vi "ScanningWaveform_v4 - Copy.vi"(0 "Vy-min":dbl, 1 "Vy-max":dbl, 2 "yPixels/tPixels":dbl, 3 "xPixels/rPixels":dbl, 4 "Vx-min":dbl, 5 "Vx-max":dbl, 6 "Drawing Mode":u16(ring) items=["Fill Rectangle", "Fill Circle", "Draw Freeform", "Fill Freeform"], 7 "Angle":dbl, 8 "Scanning Mode":u16(ring) items=["Raster", "Spiral"], 9 "AOrate":dbl, 10 "Points":cluster{"X":dbl, "Y":dbl}[](array[cluster])) -> (12 "numPixels":dbl, 13 "Y-WaveArray":dbl[](array[numeric]), 14 "P":dbl, 19 "X-WaveArray":dbl[](array[numeric]))   [LabVIEW 2013]
panel:
  out "min":dbl
  out "max":dbl
  out "Points 2":cluster{"R":dbl, "Theta":dbl}[](array[cluster])
  in  "yPixels/tPixels 2":dbl
  in  "xPixels/rPixels 2":dbl
  out "X-Y Graph":cluster{dbl[], dbl[]}(graph)
  out "flyback time (us)":dbl
  out "Y Graph":dbl[](graph)
  out "X Graph":dbl[](graph)
  out "C":dbl
  out "Sx":dbl
  out "S":dbl
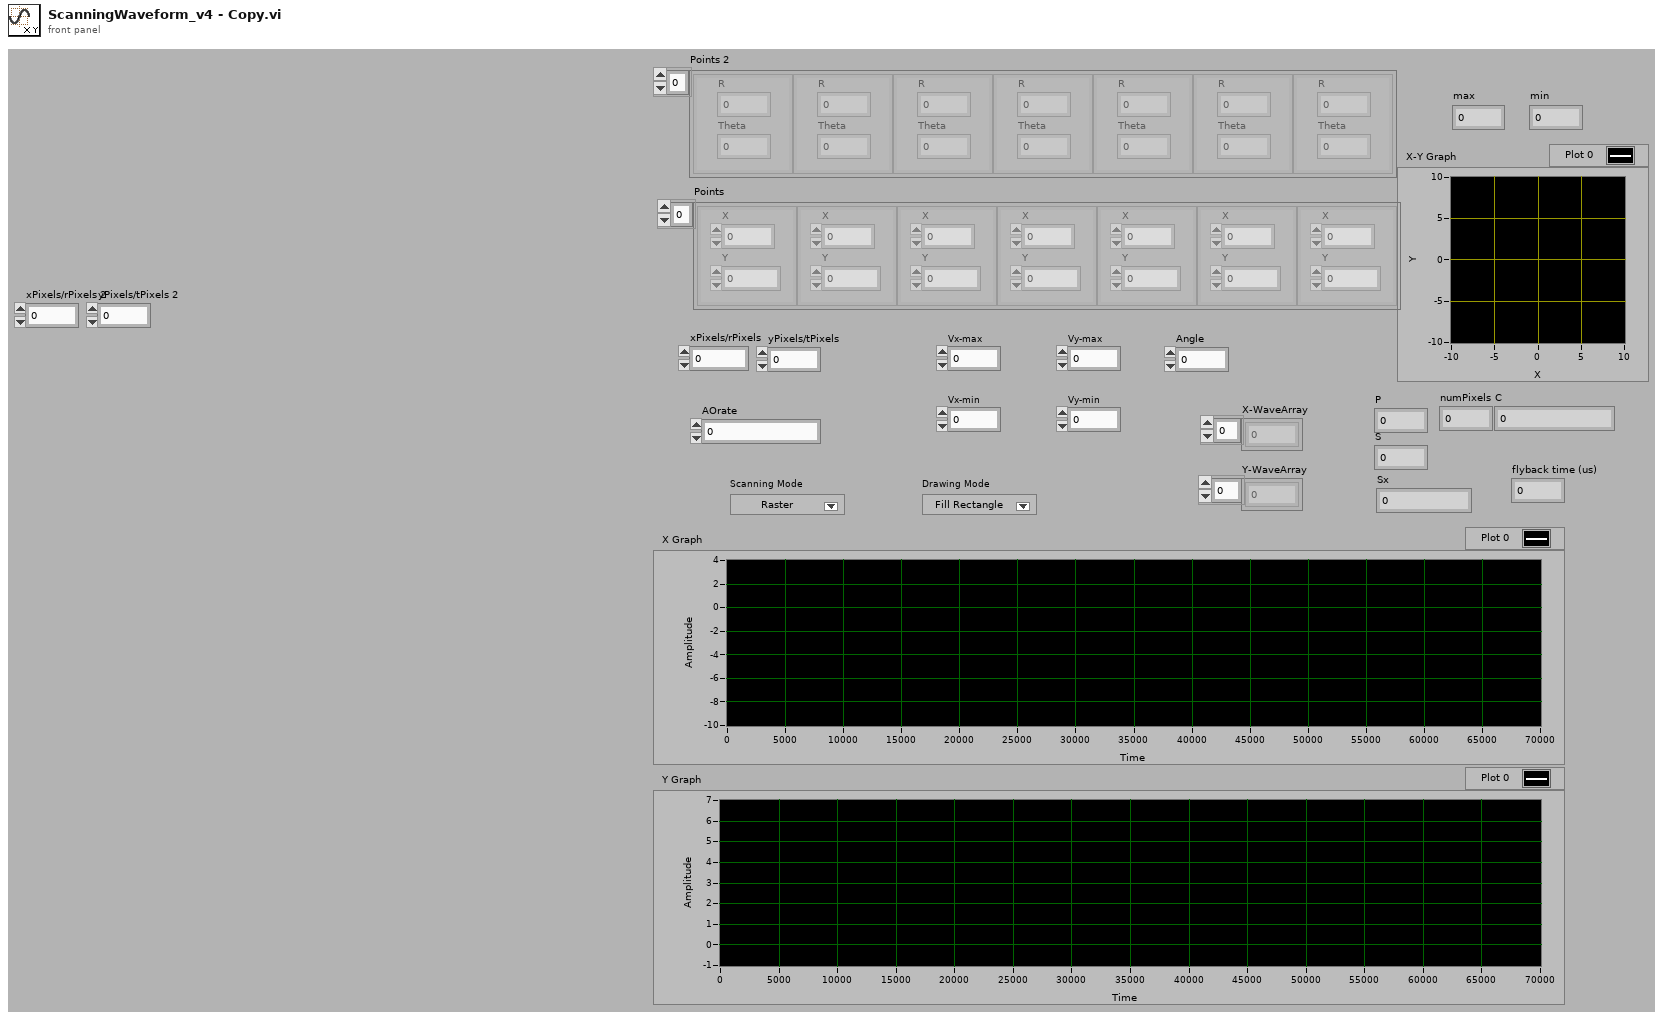
[diagram p1: front panel]
types:
  T1 = cluster{"Xpixels":i32, "Vx-min ref":dbl, "Vx-max ref":dbl, "Ypixels":i32, "Vy-min ref":dbl, "Vy-max ref":dbl, "srate":dbl, "type":string, "date":string, "time":string, "Colormap":u16, "square pixels":bool, "square matrix":bool, "Xpixels Img":i32, "Vx-min Img":dbl, "VX-max Img":dbl, "Ypixels Img":i32, "Vy-min Img":dbl, "Vy-max Img ":dbl, "autoshutter":bool, "P":dbl, "sAOxy":i32, "finite":bool, "cont":bool, "wavdet":bool, "measpoints":i32, "avpp":i32, "bufferAO":i32, "bufferAI":i32, "CH1":bool, "CH2":bool, "X":bool, "Y":bool, "timeout":dbl, "starttick":u32, "waveform":path, "Vy-ref":dbl, "Vx-ref":dbl, "refreshrate":dbl, "refreshbuffer":i32, "tt_cycles":i32, "motorref":refnum<k7>, "mirrorswitch":refnum<k7>, "sample mode":i32, "Ip":bool, "Vp":bool, "sampletreshold":dbl, "maxbufferAI":i32, "Angle Img":dbl, "Drawing Mode":u16, "Scanning Mode":u16}
  T2 = cluster{cluster{dbl, dbl}[], cluster{dbl, dbl}[]}
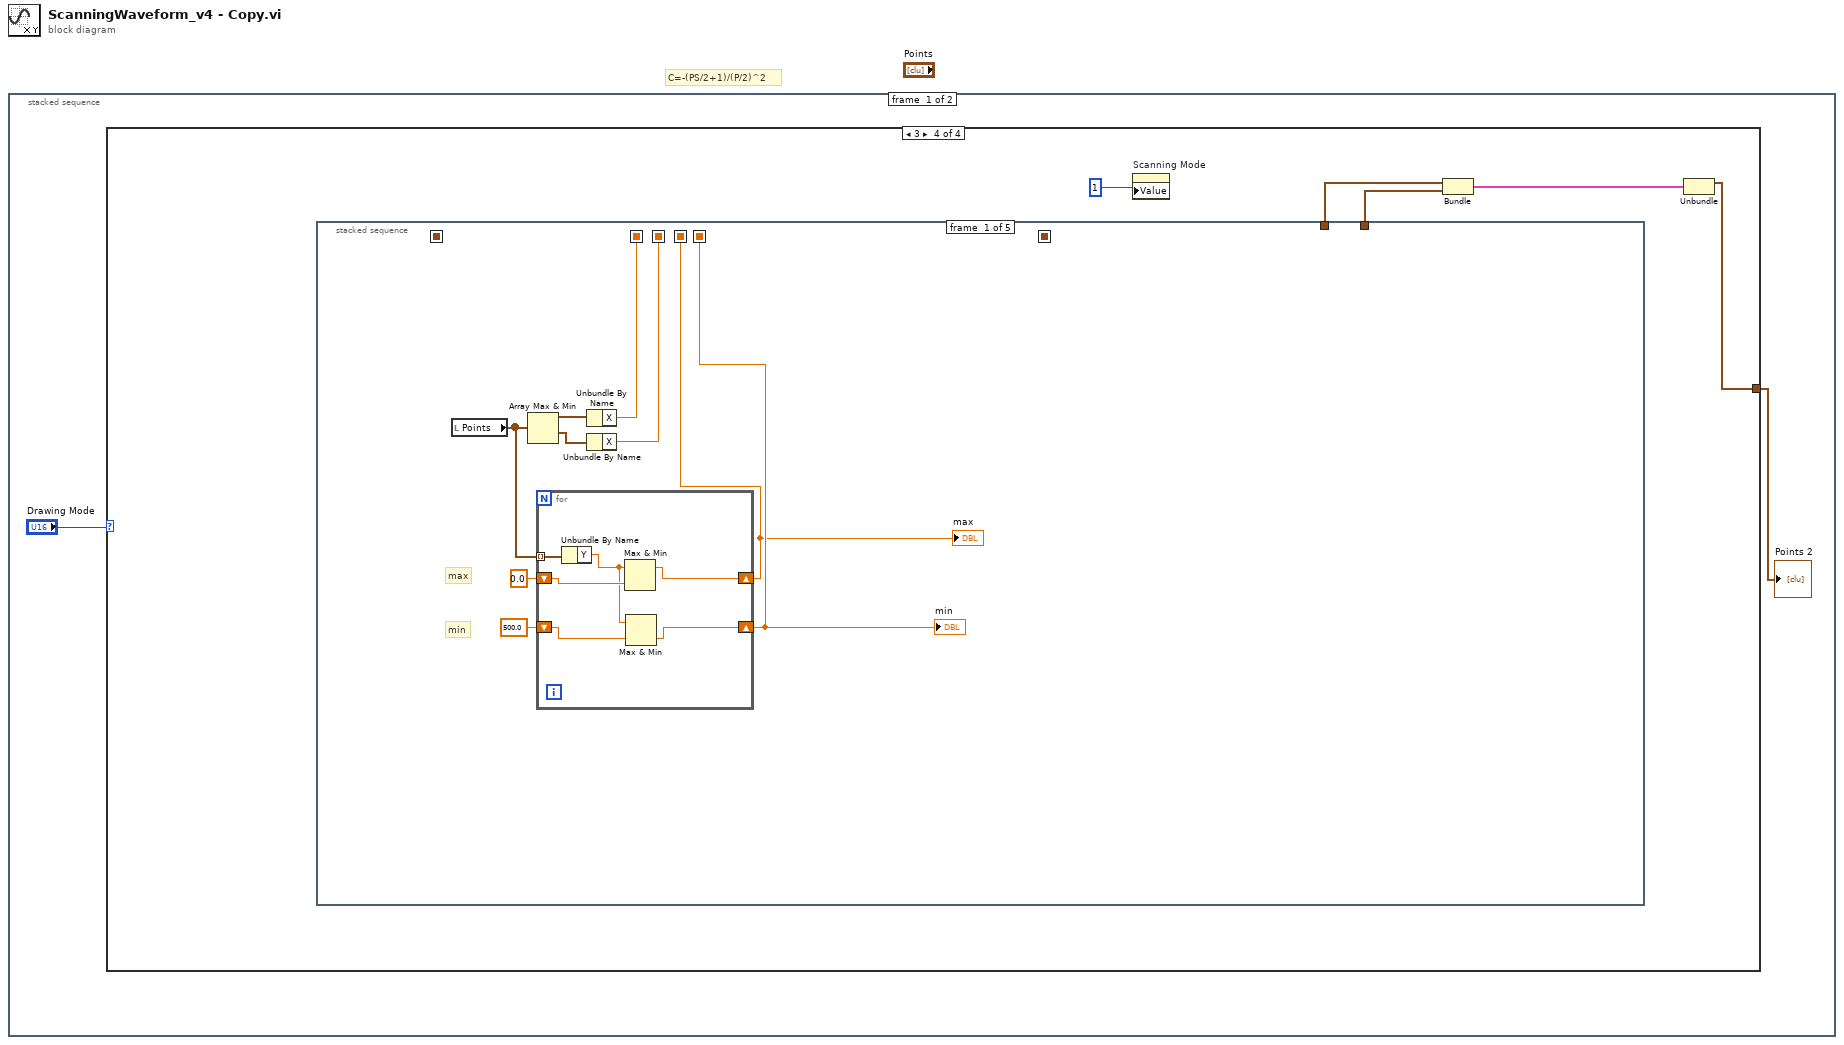
[diagram p0: block diagram]
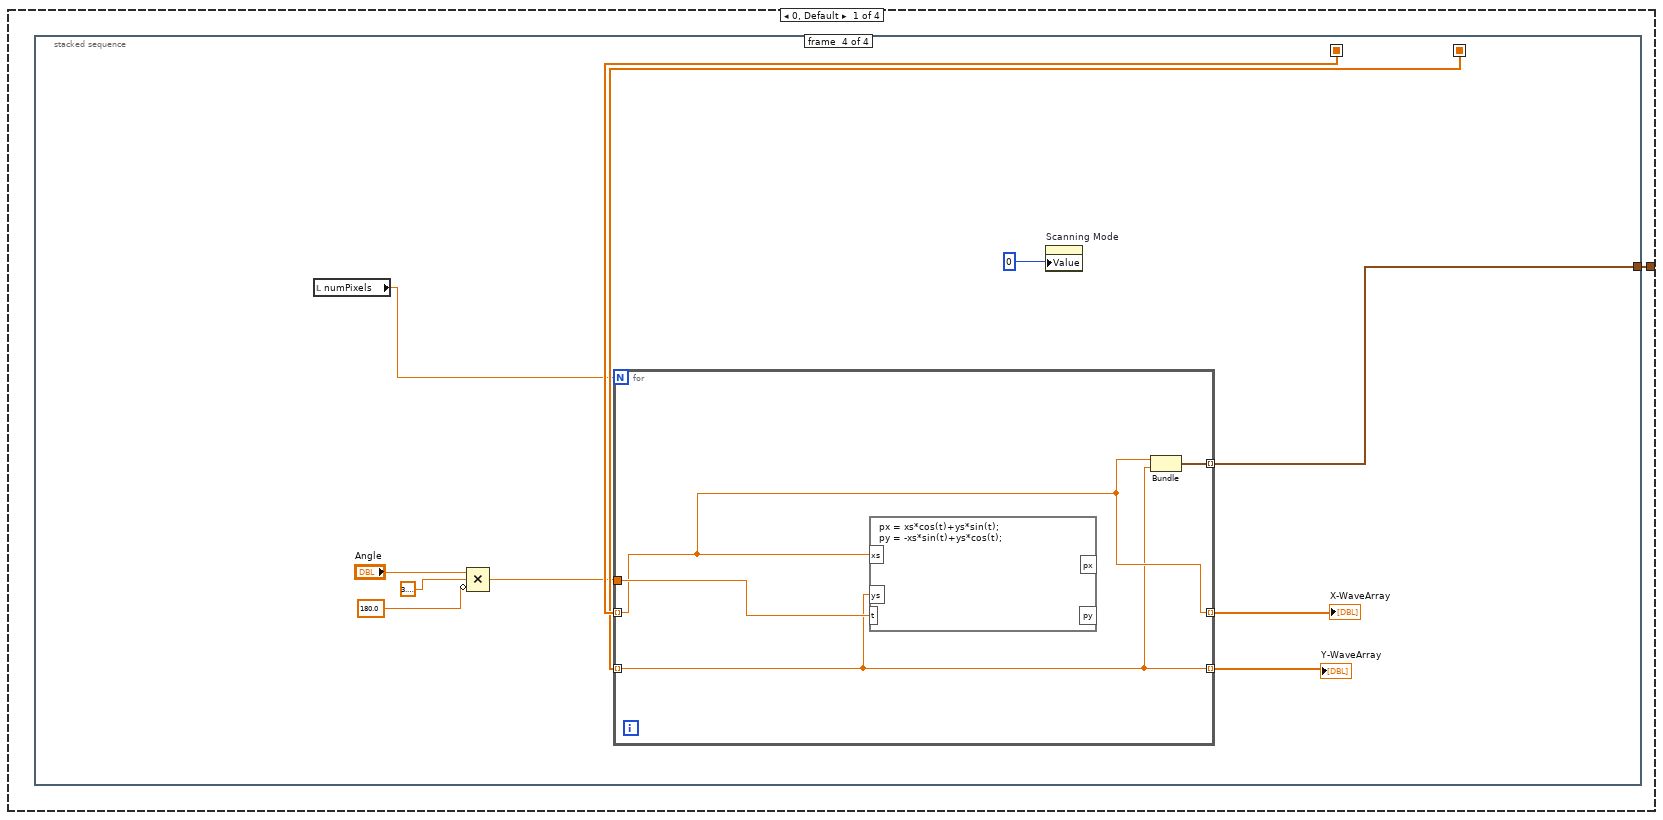
[diagram p2: hidden frame]
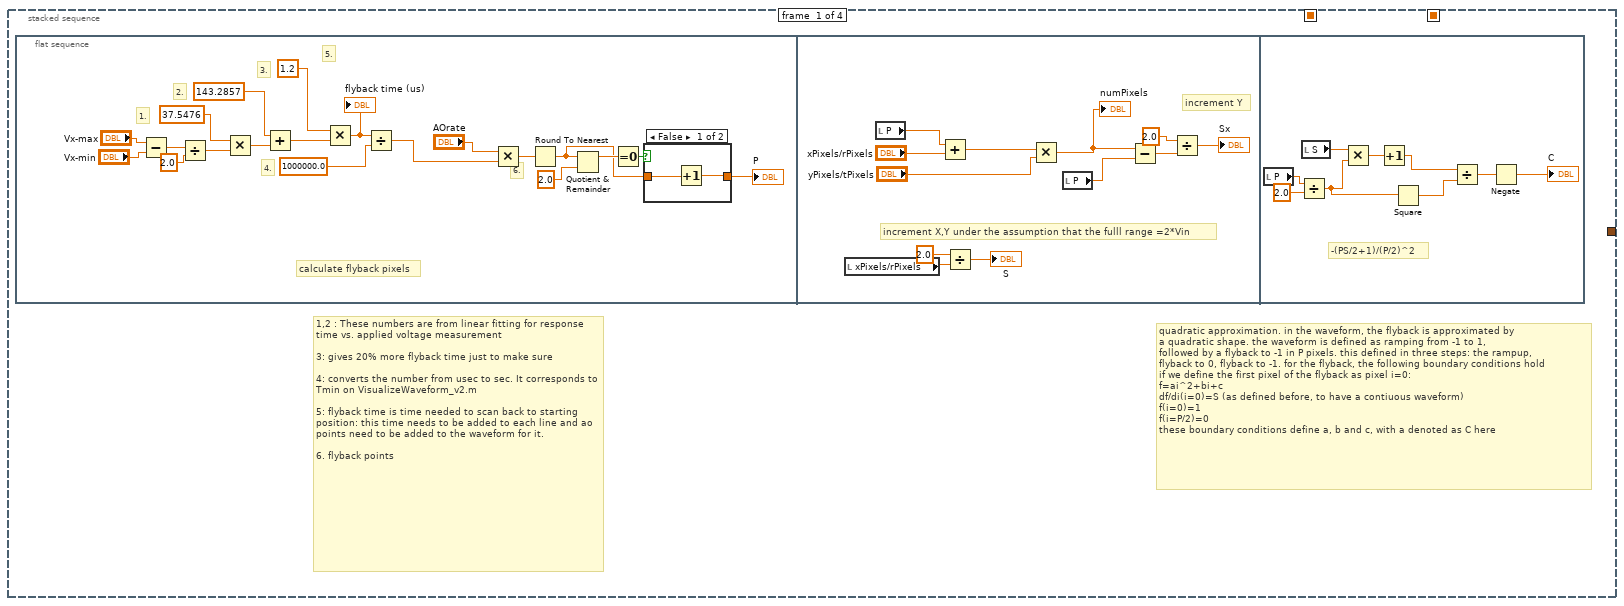
[diagram p3: hidden frame]
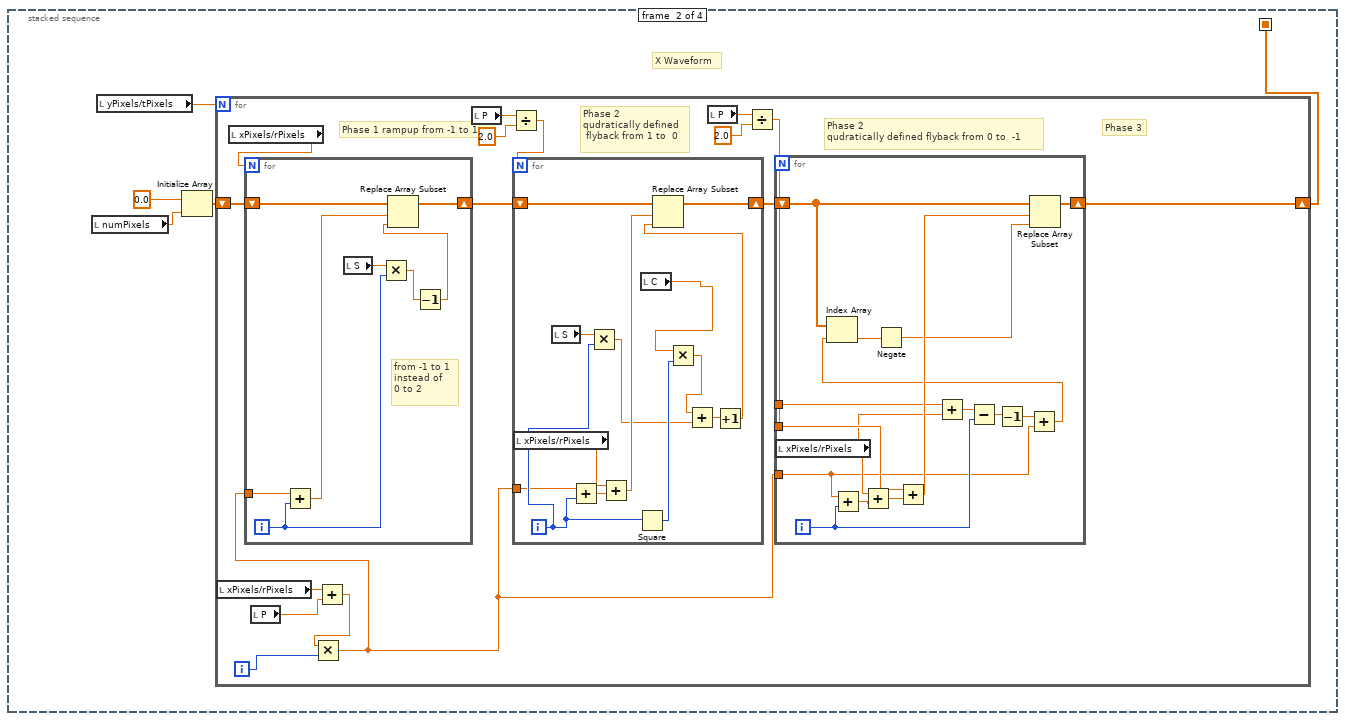
[diagram p5: hidden frame]
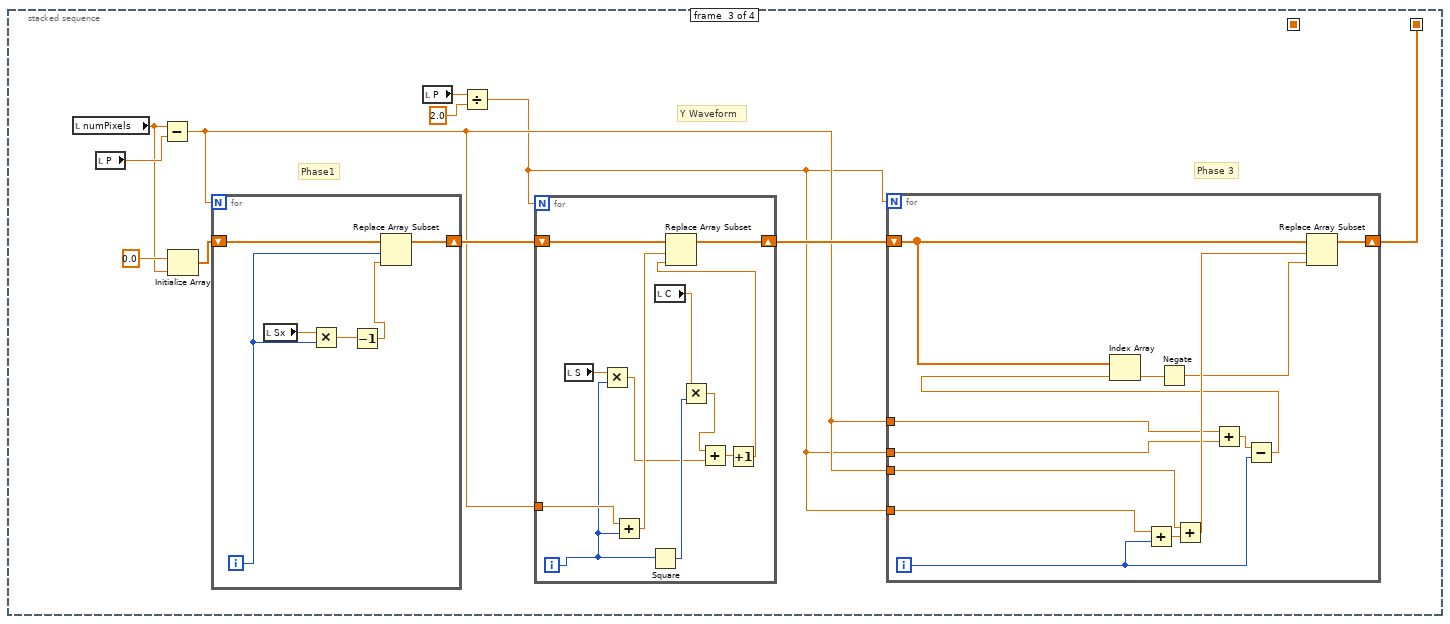
[diagram p6: hidden frame]
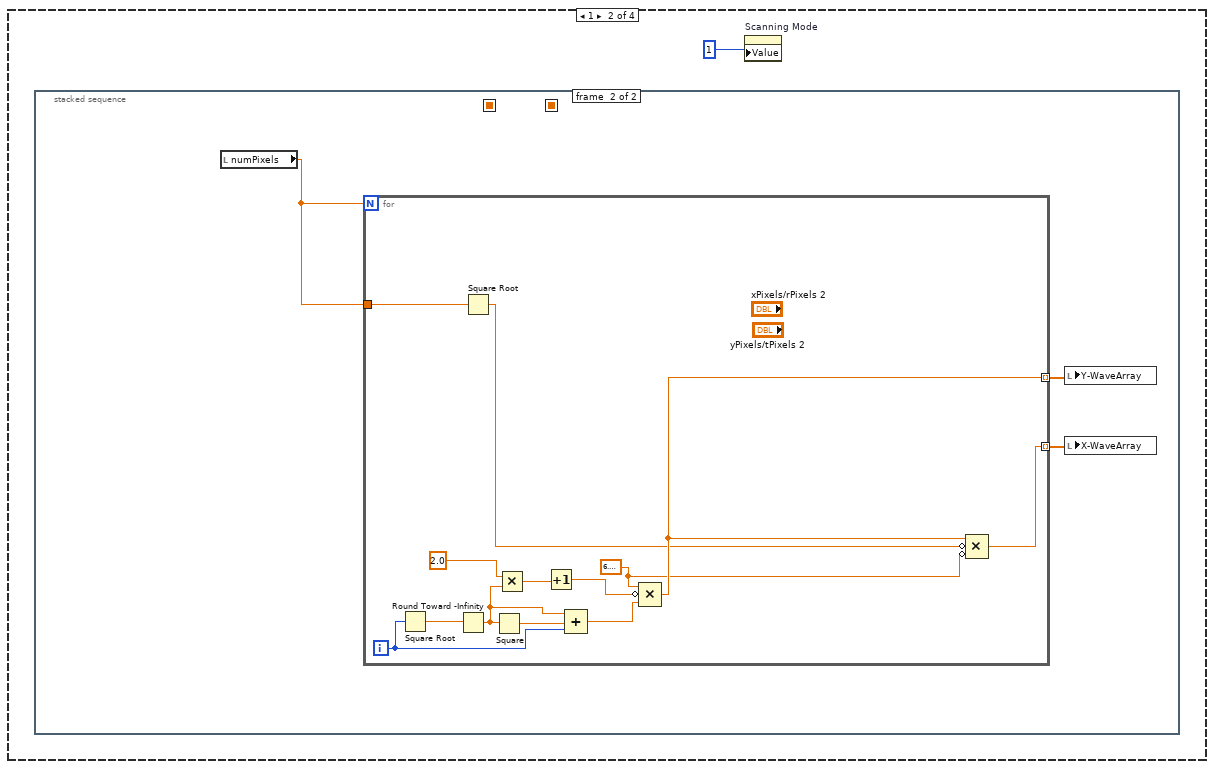
[diagram p7: hidden frame]
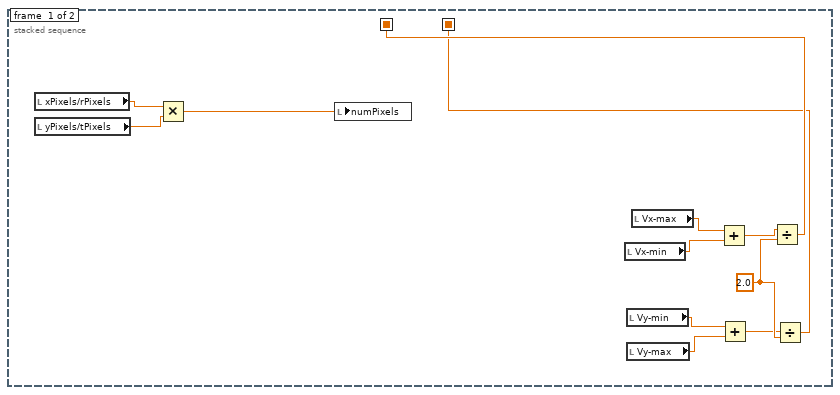
[diagram p8: hidden frame]
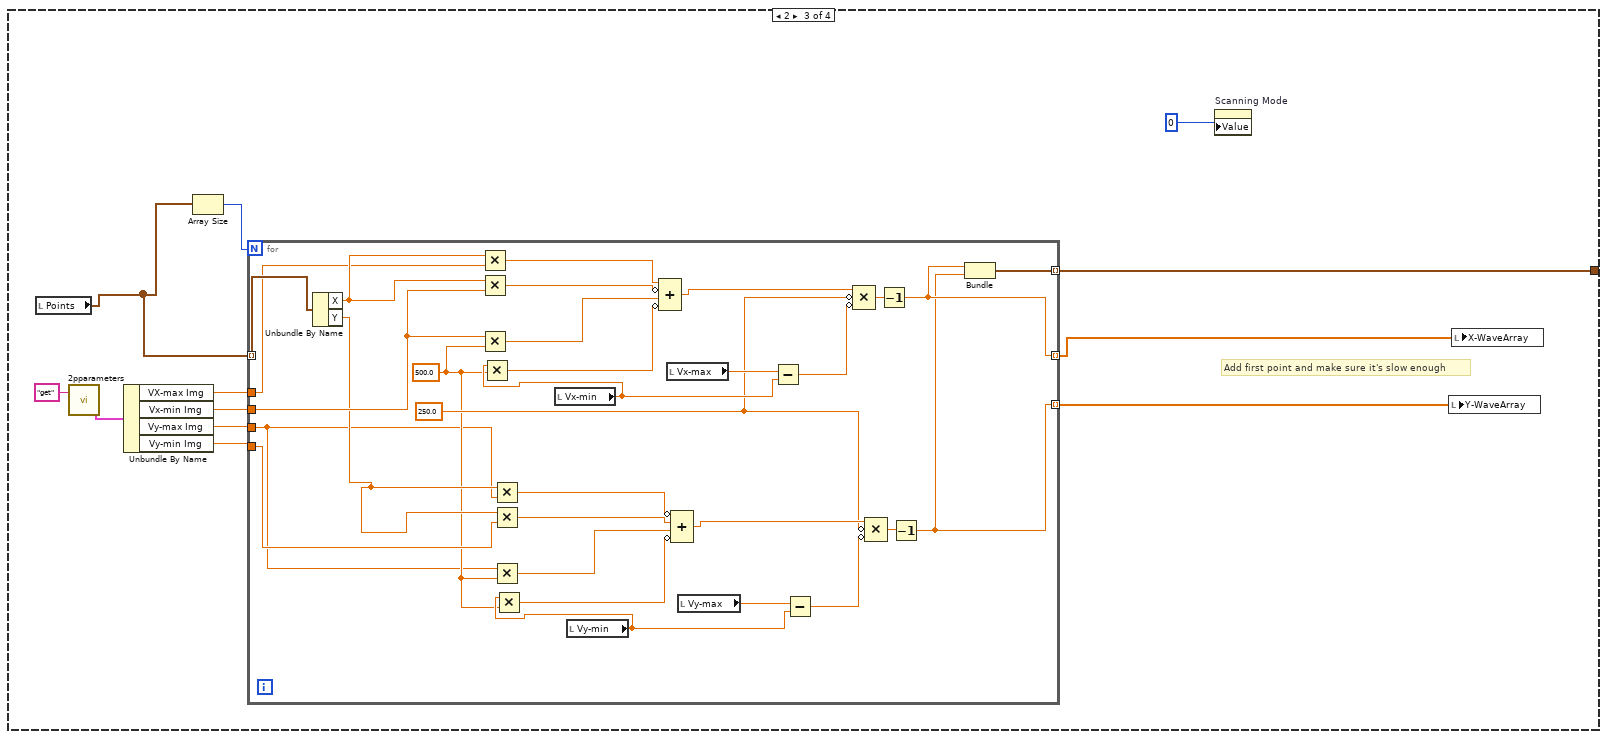
[diagram p9: hidden frame]
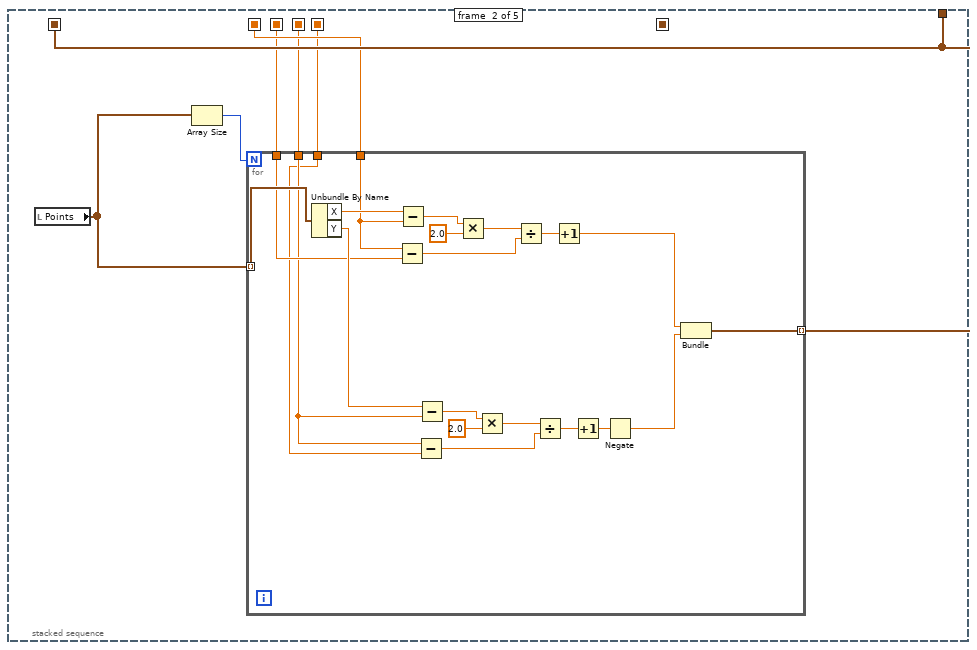
[diagram p10: hidden frame]
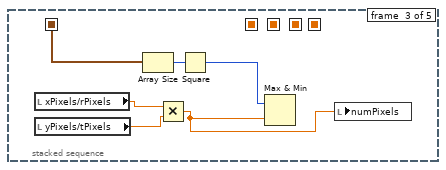
[diagram p11: hidden frame]
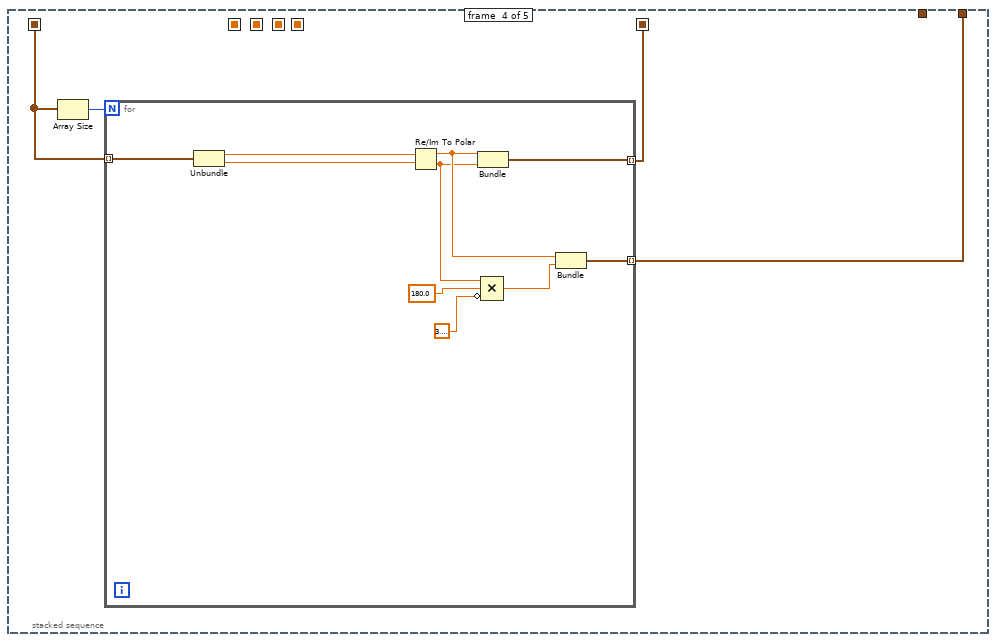
[diagram p12: hidden frame]
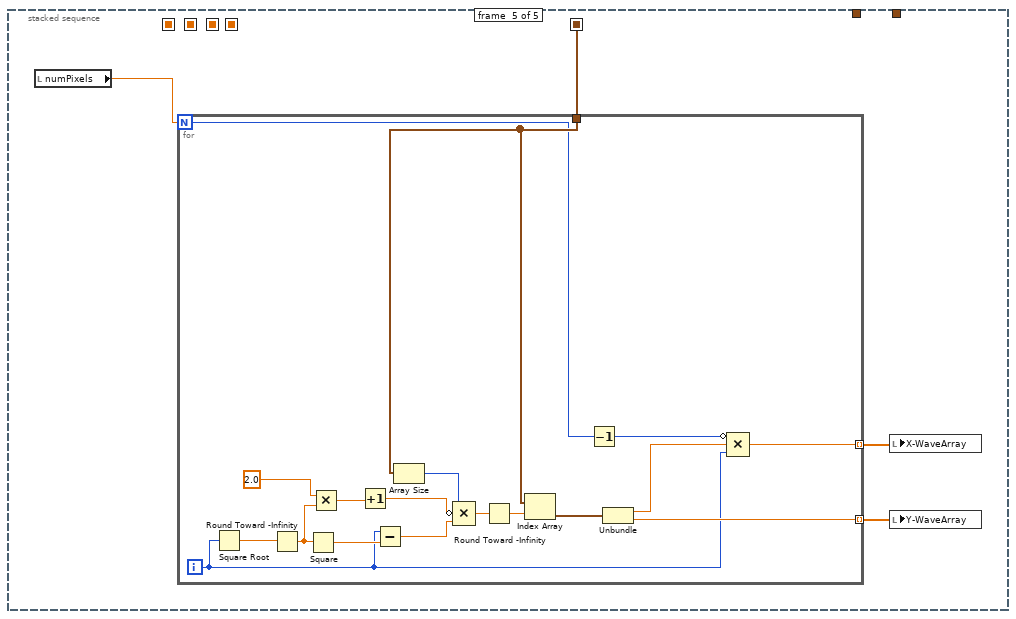
[diagram p13: hidden frame]
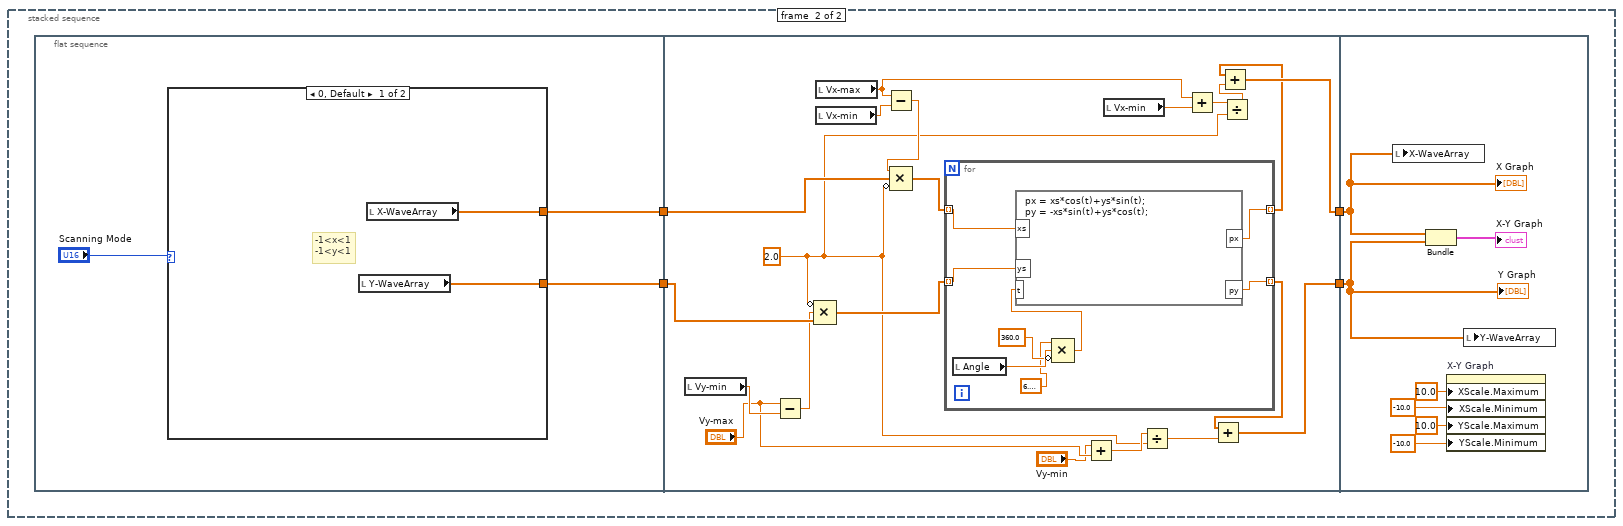
[diagram p14: hidden frame]
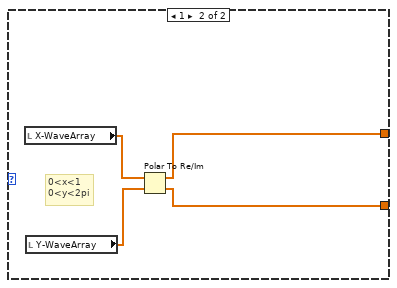
[diagram p15: hidden frame]
diagram:
  # "C=-(PS/2+1)/(P/2)^2"
  n1 = stacked-sequence {
    frame #0 {
      n2 = case shown="3" "Drawing Mode" {
        tunnel: [w3 _ w193 w236] -> w1
        frame 0, Default {
          n3 = stacked-sequence {
            seq-local: [_ w48 _ _] -> [_ _ _ w159]
            seq-local: [_ _ w107 _] -> [_ _ _ w158]
            tunnel: [_ _ _ w149] -> w3
            frame #0 {
              # "quadratic approximation. in the waveform, the flyback is approximated by\na quadratic shape. the waveform is defined as ramping from -1 to 1, \nfollowed by a flyback to -1 in P pixels. this defined in three steps: the rampup,\nflyback to 0, flyback to -1. for the flyback, the following boundary conditions hold\nif we define the first pixel of the flyback as pixel i=0:\nf=ai^2+bi+c\ndf/di(i=0)=S (as defined before, to have a contiuous waveform)\nf(i=0)=1\nf(i=P/2)=0\nthese boundary conditions define a, b and c, with a denoted as C here"
              # "1,2 : These numbers are from linear fitting for response time vs. applied voltage measurement\n\n3: gives 20% more flyback time just to make sure\n\n4: converts the number from usec to sec. It corresponds to Tmin on VisualizeWaveform_v2.m\n\n5: flyback time is time needed to scan back to starting position: this time needs to be added to each line and ao points need to be added to the waveform for it.\n\n6. flyback points"
              n4 = flat-sequence {
                frame #0 {
                  # "calculate flyback pixels"
                  # "6."
                  # "5."
                  # "4."
                  # "3."
                  # "2."
                  # "1."
                  n5 = Subtract(x="Vx-max", y="Vx-min") -> (x-y=w5:dbl)
                  n6 = Divide(x=w5, y=2.0 ("x-y")) -> (x/y=w4:dbl)
                  n7 = Multiply(x=37.5476, y=w4) -> (x*y=w21:dbl)
                  n8 = Add(x=143.2857, y=w21) -> (x+y=w19:dbl)
                  n9 = Multiply(x=1.2, y=w19) -> (x*y=w17:dbl)
                  "flyback time (us)" <- w17
                  n10 = Divide(x=w17, y=1000000.0 ("x")) -> (x/y=w15:dbl)
                  n11 = Multiply(x="AOrate", y=w15) -> (x*y=w14:dbl)
                  n12 = Round To Nearest(number=w14) -> (nearest integer value=w9:dbl)
                  n13 = Quotient & Remainder(x=w9, y=2.0) -> (x-y*floor(x/y)=w11:dbl)  [unwired: 1 out]
                  n14 = Equal To 0?(x=w11) -> (x = 0?=w12:bool)
                  n15 = case shown="False" w12 {
                    tunnel: [w24 w26] -> w10
                    tunnel: w9 -> [w25 w26]
                    frame False {
                      n16 = Increment(x=w25) -> (x+1=w24:dbl)
                    }
                    frame True {
                    }
                  }
                  "P" <- w10
                }
                frame #1 {
                  # "increment X,Y under the assumption that the fulll range =2*Vin"
                  # "increment Y"
                  n17 = local read "xPixels/rPixels"() -> (w31:dbl)
                  n18 = local read "P"() -> (w37:dbl)
                  n19 = Add(x=w37, y="xPixels/rPixels") -> (x+y=w33:dbl)
                  n20 = Divide(x=2.0, y=w31) -> (x/y=→"S":dbl)
                  n21 = Multiply(x=w33, y="yPixels/tPixels") -> (x*y=w36:dbl)
                  "numPixels" <- w36
                  n22 = local read "P"() -> (w38:dbl)
                  n23 = Subtract(x=w36, y=w38) -> (x-y=w29:dbl)
                  n24 = Divide(x=2.0, y=w29) -> (x/y=→"Sx":dbl)
                }
                frame #2 {
                  # "-(PS/2+1)/(P/2)^2"
                  n25 = local read "P"() -> (w45:dbl)
                  n26 = Divide(x=w45, y=2.0) -> (x/y=w47:dbl)
                  n27 = local read "S"() -> (w46:dbl)
                  n28 = Multiply(x=w46, y=w47) -> (x*y=w42:dbl)
                  n29 = Increment(x=w42) -> (x+1=w39:dbl)
                  n30 = Square(x=w47) -> (x^2=w43:dbl)
                  n31 = Divide(x=w39, y=w43) -> (x/y=w44:dbl)
                  n32 = Negate(x=w44) -> (-x=→"C":dbl)
                }
              }
            }
            frame #1 {
              # "X Waveform"
              n33 = local read "numPixels"() -> (w50:dbl)
              n34 = local read "yPixels/tPixels"() -> (w52:dbl)
              n35 = Initialize Array(0.0 ("element"), w50) -> (w49:dbl[])
              n36 = for {
                N: w52 -> [_]
                shift-right: [w54] -> w48
                shift-left: w49 -> [w63]
                i -> [w68]
                # "Phase 2\nqudratically defined flyback from 0 to  -1"
                # "Phase 3"
                # "Phase 2\nqudratically defined\n flyback from 1 to  0"
                # "Phase 1 rampup from -1 to 1"
                n37 = local read "xPixels/rPixels"() -> (w67:dbl)
                n38 = local read "xPixels/rPixels"() -> (w64:dbl)
                n39 = local read "P"() -> (w66:dbl)
                n40 = Add(x=w67, y=w66) -> (x+y=w65:dbl)
                n41 = Multiply(x=w65, y=w68) -> (x*y=w53:dbl)
                n42 = for {
                  N: w64 -> [_]
                  shift-right: [w102] -> w55
                  shift-left: w63 -> [w106]
                  tunnel: w53 -> [w101]
                  i -> [w103]
                  # "from -1 to 1\ninstead of\n0 to 2"
                  n43 = Add(x=w101, y=w103) -> (x+y=w105:dbl)
                  n44 = local read "S"() -> (w104:dbl)
                  n45 = Multiply(x=w104, y=w103) -> (x*y=w100:dbl)
                  n46 = Decrement(x=w100) -> (x-1=w99:dbl)
                  n47 = Replace Array Subset(array=w106, new element=w99, index=w105) -> (w102:dbl[])
                }
                n48 = local read "P"() -> (w61:dbl)
                n49 = Divide(x=w61, y=2.0) -> (x/y=w62:dbl)
                n50 = for {
                  N: w62 -> [_]
                  shift-right: [w87] -> w57
                  shift-left: w55 -> [w98]
                  tunnel: w53 -> [w86]
                  i -> [w91]
                  n51 = local read "xPixels/rPixels"() -> (w96:dbl)
                  n52 = local read "S"() -> (w92:dbl)
                  n53 = Add(x=w86, y=w91) -> (x+y=w97:dbl)
                  n54 = Multiply(x=w92, y=w91) -> (x*y=w90:dbl)
                  n55 = Add(x=w96, y=w97) -> (x+y=w95:dbl)
                  n56 = Square(x=w91) -> (x^2=w94:i32)
                  n57 = local read "C"() -> (w85:dbl)
                  n58 = Multiply(x=w85, y=w94) -> (x*y=w93:dbl)
                  n59 = Add(x=w93, y=w90) -> (x+y=w89:dbl)
                  n60 = Increment(x=w89) -> (x+1=w88:dbl)
                  n61 = Replace Array Subset(array=w98, new element=w88, index=w95) -> (w87:dbl[])
                }
                n62 = local read "P"() -> (w58:dbl)
                n63 = Divide(x=w58, y=2.0) -> (x/y=w56:dbl)
                n64 = for {
                  N: w56 -> [_]
                  tunnel: w56 -> [w82]
                  tunnel: w56 -> [w79]
                  shift-right: [w70] -> w54
                  shift-left: w57 -> [w80]
                  tunnel: w53 -> [w69]
                  i -> [w76]
                  n65 = local read "xPixels/rPixels"() -> (w78:dbl)
                  n66 = Add(x=w69, y=w76) -> (x+y=w84:dbl)
                  n67 = Add(x=w78, y=w84) -> (x+y=w83:dbl)
                  n68 = Add(x=w82, y=w83) -> (x+y=w81:dbl)
                  n69 = Add(x=w79, y=w78) -> (x+y=w77:dbl)
                  n70 = Subtract(x=w77, y=w76) -> (x-y=w75:dbl)
                  n71 = Decrement(x=w75) -> (x-1=w74:dbl)
                  n72 = Add(x=w74, y=w69) -> (x+y=w73:dbl)
                  n73 = Index Array(array=w80, index=w73) -> (element=w72:dbl)
                  n74 = Negate(x=w72) -> (-x=w71:dbl)
                  n75 = Replace Array Subset(array=w80, new element=w71, index=w81) -> (w70:dbl[])
                }
              }
            }
            frame #2 {
              # "Phase 3"
              # "Phase1"
              # "Y Waveform"
              n76 = local read "numPixels"() -> (w114:dbl)
              n77 = local read "P"() -> (w115:dbl)
              n78 = Subtract(x=w114, y=w115) -> (x-y=w109:dbl)
              n79 = Initialize Array(0.0 ("element"), w114) -> (w116:dbl[])
              n80 = for {
                N: w109 -> [_]
                shift-right: [w145] -> w111
                shift-left: w116 -> [w148]
                i -> [w146]
                n81 = local read "Sx"() -> (w147:dbl)
                n82 = Multiply(x=w147, y=w146) -> (x*y=w143:dbl)
                n83 = Decrement(x=w143) -> (x-1=w144:dbl)
                n84 = Replace Array Subset(array=w148, new element=w144, index=w146) -> (w145:dbl[])
              }
              n85 = local read "P"() -> (w113:dbl)
              n86 = Divide(x=w113, y=2.0) -> (x/y=w108:dbl)
              n87 = for {
                N: w108 -> [_]
                shift-right: [w135] -> w110
                shift-left: w111 -> [w142]
                tunnel: w109 -> [w134]
                i -> [w132]
                n88 = local read "S"() -> (w133:dbl)
                n89 = Multiply(x=w133, y=w132) -> (x*y=w138:dbl)
                n90 = Add(x=w134, y=w132) -> (x+y=w141:dbl)
                n91 = Square(x=w132) -> (x^2=w140:i32)
                n92 = local read "C"() -> (w131:dbl)
                n93 = Multiply(x=w131, y=w140) -> (x*y=w139:dbl)
                n94 = Add(x=w139, y=w138) -> (x+y=w137:dbl)
                n95 = Increment(x=w137) -> (x+1=w136:dbl)
                n96 = Replace Array Subset(array=w142, new element=w136, index=w141) -> (w135:dbl[])
              }
              n97 = for {
                N: w108 -> [_]
                shift-right: [w124] -> w107
                shift-left: w110 -> [w128]
                tunnel: w108 -> [w123]
                tunnel: w109 -> [w122]
                tunnel: w109 -> [w121]
                tunnel: w108 -> [w120]
                i -> [w118]
                n98 = Add(x=w123, y=w118) -> (x+y=w130:dbl)
                n99 = Add(x=w122, y=w130) -> (x+y=w129:dbl)
                n100 = Add(x=w121, y=w120) -> (x+y=w127:dbl)
                n101 = Subtract(x=w127, y=w118) -> (x-y=w119:dbl)
                n102 = Index Array(array=w128, index=w119) -> (element=w126:dbl)
                n103 = Negate(x=w126) -> (-x=w125:dbl)
                n104 = Replace Array Subset(array=w128, new element=w125, index=w129) -> (w124:dbl[])
              }
            }
            frame #3 {
              n105 = local read "numPixels"() -> (w153:dbl)
              n106 = Compound Arithmetic op=MULTIPLY("Angle", 3.141592653589793, invert 180.0) -> (w157:dbl)
              n107 = for {
                N: w153 -> [_]
                tunnel: w157 -> [w163]
                tunnel: w159 -> [w161] mode=indexing
                tunnel: [w161] -> w152 mode=indexing
                tunnel: w158 -> [w160] mode=indexing
                tunnel: [w160] -> w151 mode=indexing
                tunnel: [w162] -> w149 mode=indexing
                n108 = formula code="px = xs*cos(t)+ys*sin(t);\npy = -xs*sin(t)+ys*cos(t);"("xs"=w161, "ys"=w160, "t"=w163) -> ()  [unwired: 2 out]
                n109 = Bundle("element"=w161, "element"=w160) -> (w162:cluster{"element":dbl, "element":dbl})  [unwired: 1 in]
              }
              "X-WaveArray" <- w152
              "Y-WaveArray" <- w151
              n110 = property on="Scanning Mode" class="Ring (strict)"("Value"=0) -> ()  [unwired: 2 in, 2 out]
            }
          }
        }
        frame 1 {
          n111 = stacked-sequence {
            seq-local: [w166 _] -> [_ _]
            seq-local: [w170 _] -> [_ _]
            frame #0 {
              w174 = 2.0
              n112 = local read "xPixels/rPixels"() -> (w176:dbl)
              n113 = local read "yPixels/tPixels"() -> (w175:dbl)
              n114 = Multiply(x=w176, y=w175) -> (x*y=w165:dbl)
              n115 = local write "numPixels"(w165) -> ()
              n116 = local read "Vx-min"() -> (w172:dbl)
              n117 = local read "Vy-min"() -> (w169:dbl)
              n118 = local read "Vy-max"() -> (w168:dbl)
              n119 = local read "Vx-max"() -> (w173:dbl)
              n120 = Add(x=w173, y=w172) -> (x+y=w171:dbl)
              n121 = Add(x=w169, y=w168) -> (x+y=w167:dbl)
              n122 = Divide(x=w171, y=w174) -> (x/y=w170:dbl)
              n123 = Divide(x=w167, y=w174) -> (x/y=w166:dbl)
            }
            frame #1 {
              n124 = local read "numPixels"() -> (w177:dbl)
              n125 = for {
                N: w177 -> [_]
                tunnel: w177 -> [w181]
                tunnel: [w186] -> w178 mode=indexing
                tunnel: [w187] -> w179 mode=indexing
                i -> [w184]
                w182 = 6.283185307179586
                n126 = Square Root(x=w184) -> (sqrt(x)=w192:dbl)
                n127 = Round Toward -Infinity(1:w192) -> (0:w183:dbl)
                n128 = Square Root(x=w181) -> (sqrt(x)=w180:dbl)
                n129 = Square(x=w183) -> (x^2=w191:dbl)
                n130 = Multiply(x=2.0, y=w183) -> (x*y=w190:dbl)
                n131 = Increment(x=w190) -> (x+1=w189:dbl)
                n132 = Compound Arithmetic op=ADD(w183, w191, w184) -> (w185:dbl)
                n133 = Compound Arithmetic op=MULTIPLY(w182, invert w189, w185) -> (w187:dbl)
                n134 = Compound Arithmetic op=MULTIPLY(w187, invert w180, invert w182) -> (w186:dbl)
              }
              n135 = local write "Y-WaveArray"(w179) -> ()
              n136 = local write "X-WaveArray"(w178) -> ()
            }
          }
          n137 = property on="Scanning Mode" class="Ring (strict)"("Value"=1) -> ()  [unwired: 2 in, 2 out]
        }
        frame 2 {
          # "Add first point and make sure it's slow enough"
          n138 = local read "Points"() -> (w201:cluster{"X":dbl, "Y":dbl}[])
          n139 = call "2pparameters.vi"("command"="get") -> ("Params out"=w197:T1)  [unwired: 1 in]
          n140 = Unbundle By Name(w197) -> ("VX-max Img"=w199:dbl, "Vx-min Img"=w200:dbl, "Vy-max Img"=w203:dbl, "Vy-min Img"=w202:dbl)
          n141 = Array Size(array=w201) -> (size(s)=w198:i32)
          n142 = for {
            N: w198 -> [_]
            tunnel: w199 -> [w232]
            tunnel: w200 -> [w231]
            tunnel: w201 -> [w234] mode=indexing
            tunnel: w202 -> [w216]
            tunnel: w203 -> [w208]
            tunnel: [w207] -> w195 mode=indexing
            tunnel: [w206] -> w194 mode=indexing
            tunnel: [w205] -> w193 mode=indexing
            w209 = 500.0
            w215 = 250.0
            n143 = Unbundle By Name(w234) -> ("X"=w233:dbl, "Y"=w217:dbl)
            n144 = Multiply(x=w233, y=w232) -> (x*y=w213:dbl)
            n145 = Multiply(x=w233, y=w231) -> (x*y=w228:dbl)
            n146 = Multiply(x=w231, y=w209) -> (x*y=w227:dbl)
            n147 = Multiply(x=w217, y=w208) -> (x*y=w221:dbl)
            n148 = Multiply(x=w217, y=w216) -> (x*y=w222:dbl)
            n149 = Multiply(x=w208, y=w209) -> (x*y=w223:dbl)
            n150 = local read "Vx-min"() -> (w229:dbl)
            n151 = Multiply(x=w229, y=w209) -> (x*y=w226:dbl)
            n152 = local read "Vy-min"() -> (w219:dbl)
            n153 = Multiply(x=w219, y=w209) -> (x*y=w224:dbl)
            n154 = Compound Arithmetic op=ADD(w213, invert w228, w227, invert w226) -> (w211:dbl)
            n155 = local read "Vx-max"() -> (w230:dbl)
            n156 = Compound Arithmetic op=ADD(invert w221, w222, w223, invert w224) -> (w225:dbl)
            n157 = local read "Vy-max"() -> (w218:dbl)
            n158 = Subtract(x=w230, y=w229) -> (x-y=w212:dbl)
            n159 = Subtract(x=w218, y=w219) -> (x-y=w220:dbl)
            n160 = Compound Arithmetic op=MULTIPLY(w211, invert w215, invert w212) -> (w210:dbl)
            n161 = Compound Arithmetic op=MULTIPLY(w225, invert w215, invert w220) -> (w214:dbl)
            n162 = Decrement(x=w210) -> (x-1=w207:dbl)
            n163 = Decrement(x=w214) -> (x-1=w206:dbl)
            n164 = Bundle(w207, w206) -> (w205:cluster{dbl, dbl})  [unwired: 1 in]
          }
          n165 = property on="Scanning Mode" class="Ring (strict)"("Value"=0) -> ()  [unwired: 2 in, 2 out]
          n166 = local write "Y-WaveArray"(w194) -> ()
          n167 = local write "X-WaveArray"(w195) -> ()
        }
        frame 3 {
          n168 = stacked-sequence {
            seq-local: [_ _ _ w290 _] -> [_ _ _ _ w305]
            seq-local: [_ w259 _ _ _] -> [_ _ w284 w291 _]
            seq-local: [w245 _ _ _ _] -> [_ w258 _ _ _]
            seq-local: [w244 _ _ _ _] -> [_ w257 _ _ _]
            seq-local: [w242 _ _ _ _] -> [_ w256 _ _ _]
            seq-local: [w243 _ _ _ _] -> [_ w255 _ _ _]
            tunnel: [_ w259 _ _ _] -> w238
            tunnel: [_ _ _ w289 _] -> w237
            frame #0 {
              # "min"
              # "max"
              n169 = local read "Points"() -> (w246:cluster{"X":dbl, "Y":dbl}[])
              n170 = Array Max & Min(array=w246) -> (max value=w248:cluster{"X":dbl, "Y":dbl}, min value=w247:cluster{"X":dbl, "Y":dbl})  [unwired: 2 out]
              n171 = for {
                tunnel: w246 -> [w254] mode=indexing
                shift-right: [w250] -> w242
                shift-left: 0.0 -> [w253]
                shift-right: [w249] -> w243
                shift-left: 500.0 -> [w251]
                n172 = Unbundle By Name(w254) -> ("Y"=w252:dbl)
                n173 = Max & Min(x=w252, y=w253) -> (max(x,y)=w250:dbl)  [unwired: 1 out]
                n174 = Max & Min(x=w252, y=w251) -> (min(x,y)=w249:dbl)  [unwired: 1 out]
              }
              "max" <- w242
              "min" <- w243
              n175 = Unbundle By Name(w248) -> ("X"=w245:dbl)
              n176 = Unbundle By Name(w247) -> ("X"=w244:dbl)
            }
            frame #1 {
              n177 = local read "Points"() -> (w260:cluster{"X":dbl, "Y":dbl}[])
              n178 = Array Size(array=w260) -> (size(s)=w261:i32)
              n179 = for {
                N: w261 -> [_]
                tunnel: w260 -> [w282] mode=indexing
                tunnel: [w281] -> w259 mode=indexing
                tunnel: w258 -> [w267]
                tunnel: w257 -> [w266]
                tunnel: w256 -> [w265]
                tunnel: w255 -> [w264]
                n180 = Unbundle By Name(w282) -> ("X"=w269:dbl, "Y"=w268:dbl)
                n181 = Subtract(x=w267, y=w266) -> (x-y=w276:dbl)
                n182 = Subtract(x=w269, y=w267) -> (x-y=w277:dbl)
                n183 = Subtract(x=w265, y=w264) -> (x-y=w271:dbl)
                n184 = Subtract(x=w268, y=w265) -> (x-y=w272:dbl)
                n185 = Multiply(x=w277, y=2.0) -> (x*y=w278:dbl)
                n186 = Multiply(x=w272, y=2.0) -> (x*y=w273:dbl)
                n187 = Divide(x=w278, y=w276) -> (x/y=w280:dbl)
                n188 = Divide(x=w273, y=w271) -> (x/y=w274:dbl)
                n189 = Increment(x=w280) -> (x+1=w279:dbl)
                n190 = Increment(x=w274) -> (x+1=w263:dbl)
                n191 = Negate(x=w263) -> (-x=w262:dbl)
                n192 = Bundle(w279, w262) -> (w281:cluster{dbl, dbl})  [unwired: 1 in]
              }
            }
            frame #2 {
              n193 = local read "xPixels/rPixels"() -> (w288:dbl)
              n194 = local read "yPixels/tPixels"() -> (w287:dbl)
              n195 = Array Size(array=w284) -> (size(s)=w285:i32)
              n196 = Multiply(x=w288, y=w287) -> (x*y=w283:dbl)
              n197 = Square(x=w285) -> (x^2=w286:i32)
              n198 = Max & Min(x=w286, y=w283) -> ()  [unwired: 2 out]
              n199 = local write "numPixels"(w283) -> ()
            }
            frame #3 {
              n200 = Array Size(array=w291) -> (size(s)=w292:i32)
              n201 = for {
                N: w292 -> [_]
                tunnel: w291 -> [w302] mode=indexing
                tunnel: [w299] -> w290 mode=indexing
                tunnel: [w298] -> w289 mode=indexing
                n202 = Unbundle(w302) -> (w301:dbl, w300:dbl)
                n203 = Re/Im To Polar(2:w300, 3:w301) -> (0:w293:dbl, 1:w297:dbl)
                n204 = Bundle(w297, w293) -> (w299:cluster{dbl, dbl})  [unwired: 1 in]
                n205 = Compound Arithmetic op=MULTIPLY(w293, 180.0, invert 3.141592653589793) -> (w296:dbl)
                n206 = Bundle(w297, w296) -> (w298:cluster{dbl, dbl})  [unwired: 1 in]
              }
            }
            frame #4 {
              n207 = local read "numPixels"() -> (w306:dbl)
              n208 = for {
                N: w306 -> [w308]
                tunnel: w305 -> [w315]
                tunnel: [w313] -> w304 mode=indexing
                tunnel: [w312] -> w303 mode=indexing
                i -> [w310]
                n209 = Square Root(x=w310) -> (sqrt(x)=w323:dbl)
                n210 = Round Toward -Infinity(1:w323) -> (0:w321:dbl)
                n211 = Square(x=w321) -> (x^2=w322:dbl)
                n212 = Multiply(x=2.0, y=w321) -> (x*y=w320:dbl)
                n213 = Increment(x=w320) -> (x+1=w318:dbl)
                n214 = Subtract(x=w310, y=w322) -> (x-y=w317:dbl)
                n215 = Array Size(array=w315) -> (size(s)=w319:i32)
                n216 = Compound Arithmetic op=MULTIPLY(w319, invert w318, w317) -> (w311:dbl)
                n217 = Round Toward -Infinity(1:w311) -> (0:w309:dbl)
                n218 = Index Array(array=w315, index=w309) -> (element=w324:cluster{dbl, dbl})
                n219 = Decrement(x=w308) -> (x-1=w307:i32)
                n220 = Unbundle(w324) -> (w316:dbl, w313:dbl)
                n221 = Compound Arithmetic op=MULTIPLY(invert w307, w316, w310) -> (w312:dbl)
              }
              n222 = local write "X-WaveArray"(w303) -> ()
              n223 = local write "Y-WaveArray"(w304) -> ()
            }
          }
          n224 = property on="Scanning Mode" class="Ring (strict)"("Value"=u16 1) -> ()  [unwired: 2 in, 2 out]
          n225 = Bundle(w238, w237) -> (w239:T2)  [unwired: 1 in]
          n226 = Unbundle(w239) -> (w236:cluster{dbl, dbl}[])  [unwired: 1 out]
        }
      }
      "Points 2" <- w1
    }
    frame #1 {
      n227 = flat-sequence {
        tunnel: [w329] -> w328
        tunnel: [w330] -> w327
        tunnel: [w355] -> w326
        tunnel: [w356] -> w325
        tunnel: w327 -> [w357]
        tunnel: w328 -> [w358]
        tunnel: w326 -> [w372]
        tunnel: w325 -> [w371]
        frame #0 {
          n228 = case shown="0, Default" "Scanning Mode" {
            tunnel: [w333 w335] -> w329
            tunnel: [w332 w334] -> w330
            frame 0, Default {
              # "-1<x<1\n-1<y<1"
              n229 = local read "Y-WaveArray"() -> (w332:dbl[])
              n230 = local read "X-WaveArray"() -> (w333:dbl[])
            }
            frame 1 {
              # "0<x<1\n0<y<2pi"
              n231 = local read "X-WaveArray"() -> (w336:dbl[])
              n232 = local read "Y-WaveArray"() -> (w337:dbl[])
              n233 = Polar To Re/Im(2:w337, 3:w336) -> (0:w334:dbl[], 1:w335:dbl[])
            }
          }
        }
        frame #1 {
          w340 = 2.0
          n234 = local read "Vy-min"() -> (w351:dbl)
          n235 = Subtract(x="Vy-max", y=w351) -> (x-y=w353:dbl)
          n236 = Compound Arithmetic op=MULTIPLY(invert w340, w353, w357) -> (w349:dbl[])
          n237 = local read "Vx-max"() -> (w346:dbl)
          n238 = local read "Vx-min"() -> (w354:dbl)
          n239 = Subtract(x=w346, y=w354) -> (x-y=w352:dbl)
          n240 = Compound Arithmetic op=MULTIPLY(w352, w358, invert w340) -> (w350:dbl[])
          n241 = for {
            tunnel: [w366] -> w348 mode=indexing
            tunnel: [w365] -> w347 mode=indexing
            tunnel: w350 -> [w364] mode=indexing
            tunnel: w349 -> [w363] mode=indexing
            n242 = local read "Angle"() -> (w362:dbl)
            n243 = Compound Arithmetic op=MULTIPLY(6.283185307179586, w362, invert 360.0) -> (w359:dbl)
            n244 = formula code="px = xs*cos(t)+ys*sin(t);\npy = -xs*sin(t)+ys*cos(t);"("xs"=w364, "ys"=w363, "t"=w359) -> ("px"=w366:dbl, "py"=w365:dbl)
          }
          n245 = Add(x="Vy-min", y="Vy-max") -> (x+y=w341:dbl)
          n246 = local read "Vx-min"() -> (w345:dbl)
          n247 = Divide(x=w341, y=w340) -> (x/y=w342:dbl)
          n248 = Add(x=w346, y=w345) -> (x+y=w344:dbl)
          n249 = Add(x=w347, y=w342) -> (x+y=w356:dbl[])
          n250 = Divide(x=w344, y=w340) -> (x/y=w343:dbl)
          n251 = Add(x=w348, y=w343) -> (x+y=w355:dbl[])
        }
        frame #2 {
          n252 = local write "X-WaveArray"(w372) -> ()
          n253 = Bundle(w372, w371) -> (→"X-Y Graph":cluster{dbl[], dbl[]})  [unwired: 1 in]
          n254 = property on="X-Y Graph" class="XYGraph (strict)"("XScale.Maximum"=10.0 ("X Scale.Range:Maximum"), "XScale.Minimum"=-10.0 ("X Scale.Range:Minimum"), "YScale.Maximum"=10.0 ("Y Scale.Range:Maximum"), "YScale.Minimum"=-10.0 ("Y Scale.Range:Minimum")) -> ()  [unwired: 2 in, 2 out]
          n255 = local write "Y-WaveArray"(w371) -> ()
          "X Graph" <- w372
          "Y Graph" <- w371
        }
      }
    }
  }
